vi "海流计写数据库.vi"(10 "Tabe Name":string="海流计", 11 "data":T1) -> ()   [LabVIEW 2016, in "AADI5400.lvlib"]
uses:
  AADI5400.lvlib
panel:
  out "错误输出":errorcluster
  in  "错误输入（无错误）":errorcluster
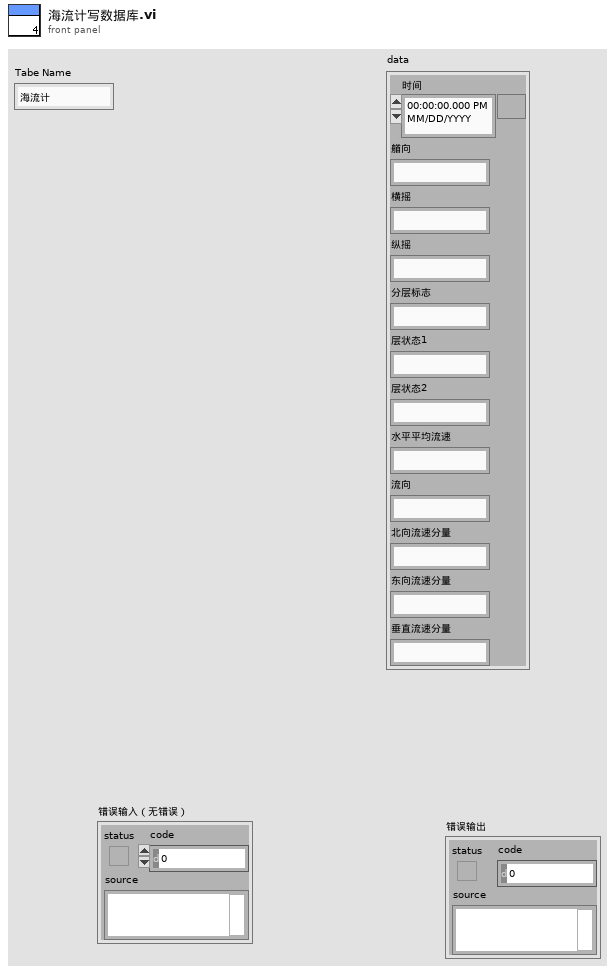
[diagram p1: front panel]
types:
  T1 = cluster{"时间":timestamp, "艏向":string, "横摇":string, "纵摇":string, "分层标志":string, "层状态1":string, "层状态2":string, "水平平均流速":string, "流向":string, "北向流速分量":string, "东向流速分量":string, "垂直流速分量":string}
  T2 = typedef "LVDateTimeRec.ctl" = cluster{"秒数的小数部分":dbl, "秒":i32, "分":i32, "时":i32, "日":i32, "月":i32, "年":i32, "天数（周）":i32, "天数（年）":i32, "DST":i32}
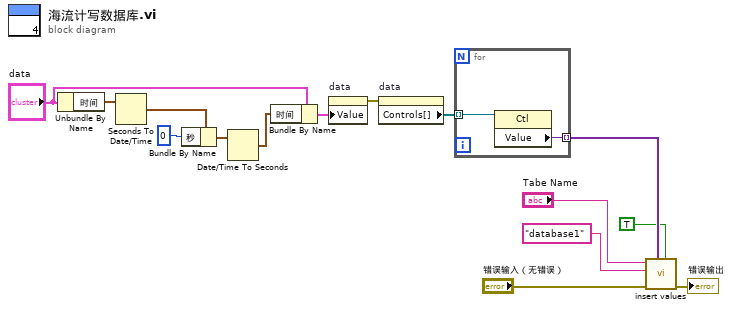
[diagram p0: block diagram]
diagram:
  n1 = Unbundle By Name("data") -> ("时间"=w8:timestamp)
  n2 = Seconds To Date/Time(time stamp (now)=w8) -> (date time rec=w7:T2)  [unwired: 1 in]
  n3 = Bundle By Name(cluster=w7, "秒"=0) -> (w5:T2)
  n4 = Date/Time To Seconds(2:w5) -> (0:w3:timestamp)  [unwired: 1 in]
  n5 = Bundle By Name(cluster="data", "时间"=w3) -> (w2:T1)
  n6 = property on="data" class="Clust (严格)"("Value"=w2) -> (error out=w1:errorcluster)  [unwired: 2 in, 1 out]
  n7 = property on="data" class="Clust (严格)"(error in=w1) -> ("Controls[]"=w9:refnum<vi>[])  [unwired: 1 in, 2 out]
  n8 = for {
    tunnel: w9 -> [w17] mode=indexing
    tunnel: [w16] -> w15 mode=indexing
    n9 = property class="Ctl"(reference=w17) -> ("Value"=w16:variant)  [unwired: 1 in, 2 out]
  }
  n10 = call "insert values.vi"("是否创建唯一键"=TRUE, "data"=w15, "错误输入（无错误）"="错误输入（无错误）", "database"="database1", "Tabe Name"="Tabe Name") -> ("错误输出"=→"错误输出":errorcluster)  [unwired: 6 in]
